vi "meth.RunChunk.vi"(0 "GLue in":refnum<class "class.GLue.lvclass">, 2 "Script":string, 7 "Data in":variant, 11 "error in":errorcluster, 13 "Name":string="Chunk") -> (4 "GLue out":refnum<class "class.GLue.lvclass">, 8 "Data out":variant, 15 "error out":errorcluster)   [LabVIEW 2014, in "GLue.lvlib" / "class.GLue.lvclass"]
uses:
  class.GLue.lvclass
  class.GLue.lvclass/class.GLue.ctl
  wrap.GetStatus.vi
  wrap.ReInit.vi
  vi.ClearLVData.vi
  meth.PushErrorState.vi
  vi.ModuleExecute.vi
  wrap.PushBool.vi
  wrap.PushString.vi
  meth.PushLVData.vi
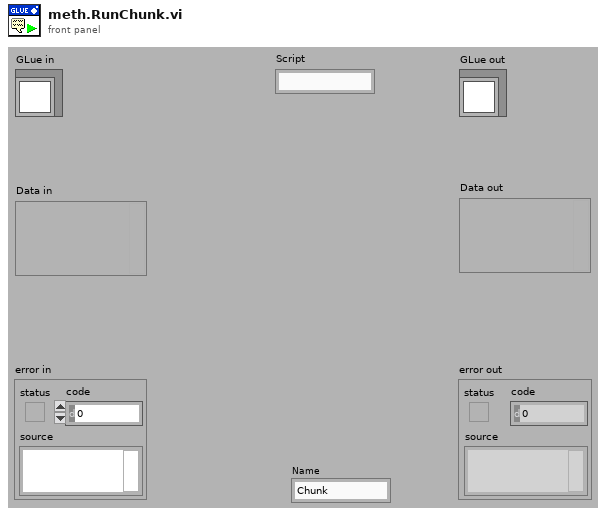
[diagram p1: front panel]
types:
  T1 = cluster{"EventRef":refnum<event-registration>, "Reader":cluster{"StreamReader":refnum<vi>, "UserData":variant}}
  T2 = typedef "GLue.lvlib/class.GLue.lvclass/typedef.Types.ctl" = enum16{"Nil", "Bool", "LightUserData", "Number", "String", "Table", "Function", "UserData", "Thread"}
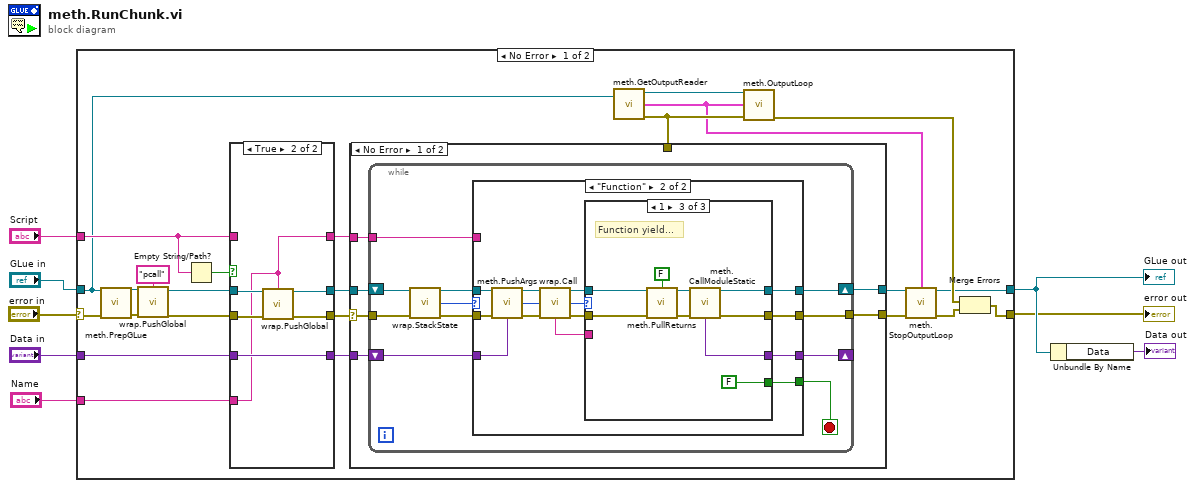
[diagram p0: block diagram]
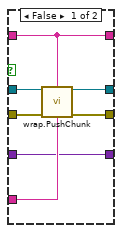
[diagram p2: hidden frame]
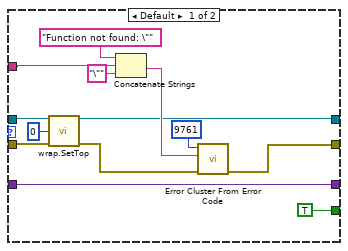
[diagram p3: hidden frame]
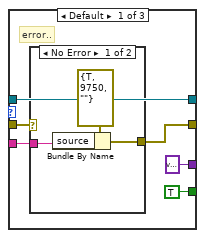
[diagram p4: hidden frame]
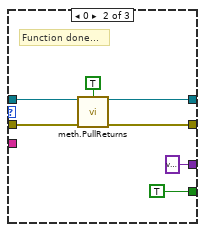
[diagram p6: hidden frame]
diagram:
  n1 = case shown="No Error" "error in" {
    selector: "error in" -> [w32 w119]
    tunnel: [w14 w119] -> w1
    tunnel: [w12 w118] -> w2
    tunnel: "GLue in" -> [w18 w118]
    tunnel: "Data in" -> [w23 _]
    tunnel: "Script" -> [w20 _]
    tunnel: "Name" -> [w24 _]
    frame No Error {
      n2 = call "meth.PrepGLue.vi"("class.GLue in"=w18, "error in"=w32) -> ("class.GLue out"=w26:refnum<class "class.GLue.lvclass">, "error out"=w25:errorcluster)  [unwired: 12 in]
      n3 = call "wrap.PushGlobal.vi"("class.GLue in"=w26, "Name"="pcall", "error in (no error)"=w25) -> ("class.GLue out"=w27:refnum<class "class.GLue.lvclass">, "error out"=w28:errorcluster)  [unwired: 11 in]
      n4 = Empty String/Path?(string/path=w20) -> (empty?=w19:bool)
      n5 = case shown="True" w19 {
        tunnel: [w39 w42] -> w31
        tunnel: [w38 w43] -> w30
        tunnel: w28 -> [w37 w45]
        tunnel: w27 -> [w36 w44]
        tunnel: w24 -> [w35 w40]
        tunnel: w23 -> [w34 w41]
        tunnel: [w34 w41] -> w22
        tunnel: w20 -> [w33 _]
        tunnel: [w33 w40] -> w21
        frame False {
          n6 = call "wrap.PushChunk.vi"("class.GLue in"=w36, "Script"=w33, "error in (no error)"=w37, "Name"=w35) -> ("class.GLue out"=w39:refnum<class "class.GLue.lvclass">, "error out"=w38:errorcluster)  [unwired: 10 in]
        }
        frame True {
          n7 = call "wrap.PushGlobal.vi"("class.GLue in"=w44, "Name"=w40, "error in (no error)"=w45) -> ("class.GLue out"=w42:refnum<class "class.GLue.lvclass">, "error out"=w43:errorcluster)  [unwired: 11 in]
        }
      }
      n8 = call "meth.GetOutputReader.vi"("class.GLue in"=w18) -> ("class.GLue out"=w10:refnum<class "class.GLue.lvclass">, "ReaderContext"=w9:T1, "error out"=w11:errorcluster)  [unwired: 12 in]
      n9 = case shown="No Error" w30 {
        selector: w30 -> [w48 w117]
        tunnel: w22 -> [w51 _]
        tunnel: [w47 w116] -> w16
        tunnel: [w46 w117] -> w17
        tunnel: w21 -> [w50 _]
        tunnel: w31 -> [w49 w116]
        tunnel: w11 -> [_ _]
        frame No Error {
          n10 = while {
            tunnel: [w57] -> w46
            shift-right: [w56] -> w47
            shift-left: w49 -> [w52]
            shift-right: [w55] -> _
            shift-left: w51 -> [w58]
            tunnel: w50 -> [w54]
            tunnel: w48 -> [w53]
            stop <- w60 stop-if-true
            n11 = call "wrap.StackState.vi"("class.GLue in"=w52, "error in (no error)"=w53) -> ("class.GLue out"=w59:refnum<class "class.GLue.lvclass">, "TopType"=w62:T2, "error out"=w61:errorcluster)  [unwired: 10 in, 1 out]
            n12 = case shown="\"Function\"" w62 {
              tunnel: w61 -> [w66 w89]
              tunnel: [TRUE w80] -> w60
              tunnel: w59 -> [w67 w88]
              tunnel: w58 -> [w74 w87]
              tunnel: [w73 w79] -> w57
              tunnel: [w65 w78] -> w56
              tunnel: [w74 w77] -> w55
              tunnel: w54 -> [w70 _]
              frame Default {
                n13 = call "wrap.SetTop.vi"("class.GLue in"=w67, "Index"=0, "error in (no error)"=w66) -> ("class.GLue out"=w65:refnum<class "class.GLue.lvclass">, "error out"=w64:errorcluster)  [unwired: 11 in]
                n14 = Concatenate Strings("Function not found: \"" ("error message (\"\")"), w70, "\"" ("string")) -> (w68:string)
                n15 = call <vilib>:"Error Cluster From Error Code.vi"("error in (no error)"=w64, "error message (\"\")"=w68, "error code (0)"=9761) -> ("error out"=w73:errorcluster)  [unwired: 6 in]
              }
              frame "Function" {
                n16 = call "meth.PushArgs.vi"("class.GLue in"=w88, "error in (no error)"=w89, "Variant in"=w87) -> ("class.GLue out"=w85:refnum<class "class.GLue.lvclass">, "NumArgs"=w84:i32, "error out"=w86:errorcluster)  [unwired: 10 in]
                n17 = call "wrap.Call.vi"("class.GLue in"=w85, "NumArgs"=w84, "error in (no error)"=w86) -> ("class.GLue out"=w82:refnum<class "class.GLue.lvclass">, "Return"=w83:i32, "ErrString"=w76:string, "error out"=w81:errorcluster)  [unwired: 9 in]
                n18 = case shown="1" w83 {
                  tunnel: w82 -> [w94 w105 w111]
                  tunnel: w81 -> [w91 w106 w107]
                  tunnel: [TRUE TRUE FALSE] -> w80
                  tunnel: [w90 w103 w114] -> w79
                  tunnel: [w94 w102 w113] -> w78
                  tunnel: [variant ("Data Out") variant ("Data Out") w115] -> w77
                  tunnel: w76 -> [w92 _ _]
                  frame Default {
                    # "error.."
                    n19 = case shown="No Error" w91 {
                      selector: w91 -> [_ w99]
                      tunnel: w92 -> [w97 _]
                      tunnel: [w96 w99] -> w90
                      frame No Error {
                        n20 = Bundle By Name(cluster=errorcluster {"status"=TRUE, "code"=9750, "source"=""} ("error out"), "source"=w97) -> (w96:errorcluster)
                      }
                      frame Error {
                      }
                    }
                  }
                  frame 0 {
                    # "Function done..."
                    n21 = call "meth.PullReturns.vi"("class.GLue in"=w105, "ScriptReturn"=TRUE, "error in"=w106) -> ("class.GLue out"=w102:refnum<class "class.GLue.lvclass">, "error out"=w103:errorcluster)  [unwired: 11 in]
                  }
                  frame 1 {
                    # "Function yield..."
                    n22 = call "meth.PullReturns.vi"("class.GLue in"=w111, "ScriptReturn"=FALSE, "error in"=w107) -> ("class.GLue out"=w109:refnum<class "class.GLue.lvclass">, "error out"=w110:errorcluster)  [unwired: 11 in]
                    n23 = call "meth.CallModuleStatic.vi"("GLue in"=w109, "error in"=w110) -> ("GLue out"=w113:refnum<class "class.GLue.lvclass">, "Data Out"=w115:variant, "error out"=w114:errorcluster)  [unwired: 11 in]
                  }
                }
              }
            }
          }
        }
        frame Error {
        }
      }
      n24 = call "meth.OutputLoop.vi"("class.GLue in"=w10, "ReaderContext in"=w9, "error in"=w11) -> ("error out"=w13:errorcluster)  [unwired: 11 in, 1 out]
      n25 = call "meth.StopOutputLoop.vi"("class.GLue in"=w16, "ReaderContext in"=w9, "error in"=w17) -> ("class.GLue out"=w12:refnum<class "class.GLue.lvclass">, "error out"=w15:errorcluster)  [unwired: 11 in]
      n26 = Merge Errors(w13, w15) -> (w14:errorcluster)
    }
    frame Error {
    }
  }
  "error out" <- w1
  "GLue out" <- w2
  n27 = Unbundle By Name(w2) -> ("Data"=→"Data out":variant)
